vi "broadcastFAFreezeSensorValues.vi"(8 "error in (no error)":errorcluster, 10 "ModbusBuffer in":refnum<class "ModbusBuffer.lvclass">, 11 "ILCCommunications in":refnum<class "ILCCommunications.lvclass">) -> (0 "error out":errorcluster, 2 "ModbusBuffer out":refnum<class "ModbusBuffer.lvclass">, 3 "ILCCommunications out":refnum<class "ILCCommunications.lvclass">)   [LabVIEW 2016, in "ILCCommunications.lvclass"]
uses:
  ILCCommunications.lvclass
  Common_RT_Modbus/ModbusBuffer/ModbusBuffer.lvclass
  ILCCommunications.lvclass/ILCCommunications.ctl
  Common_RT_FAILC/FAILC/FAILC.lvclass/FAILC.ctl
  Common_RT_ILC/ILC/ILC.lvclass/ILC.ctl
  Common_RT_Modbus/ModbusBuffer/ModbusBuffer.lvclass/ModbusBuffer.ctl
  Common_RT_Modbus/ModbusBuffer/writeHeader.vi
  Common_RT_Modbus/ModbusBuffer/writeU8.vi
  Common_RT_Modbus/ModbusBuffer/writeCRC.vi
  Common_RT_Modbus/ModbusBuffer/writeEndOfFrame.vi
  Common_RT_Modbus/ModbusBuffer/writeDelay.vi
  Common_RT_ILC/ILC/getILCData.vi
  Common_RT_Modbus/ModbusBuffer/writeByteInstruction.vi
  Common_RT_Modbus/ModbusBuffer/calculateCRC.vi
  Common_RT_FAILC/FAILC/FAILC.lvclass
  D:/Code/ts_M1M3Support/Common_RT_ILC/ILC/ILC.lvclass
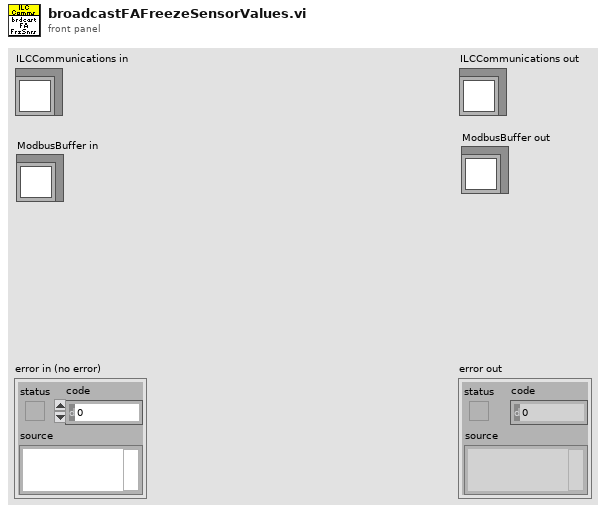
[diagram p1: front panel]
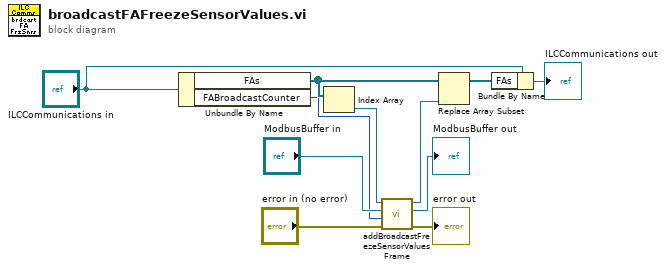
[diagram p0: block diagram]
diagram:
  n1 = Unbundle By Name("ILCCommunications in") -> ("FAs"=w11:refnum<class "FAILC.lvclass">[], "FABroadcastCounter"=w5:u8)
  n2 = Index Array(array=w11) -> (element=w7:refnum<class "FAILC.lvclass">)  [unwired: 1 in]
  n3 = call "addBroadcastFreezeSensorValuesFrame.vi"("error in (no error)"="error in (no error)", "BroadcastCounter"=w5, "ModbusBuffer in"="ModbusBuffer in", "FAILC in"=w7) -> ("error out"=→"error out":errorcluster, "ModbusBuffer out"=→"ModbusBuffer out":refnum<class "ModbusBuffer.lvclass">, "FAILC out"=w1:refnum<class "FAILC.lvclass">)  [unwired: 5 in]
  n4 = Replace Array Subset(array=w11, new element=w1) -> (w9:refnum<class "FAILC.lvclass">[])  [unwired: 1 in]
  n5 = Bundle By Name(cluster="ILCCommunications in", "FAs"=w9) -> (→"ILCCommunications out":refnum<class "ILCCommunications.lvclass">)
